vi "Read Display Name.vi"(8 "error in (no error)":errorcluster, 11 "Task in":refnum<class "Task.lvclass">) -> (0 "error out":errorcluster, 2 "Display Name":string, 3 "Task out":refnum<class "Task.lvclass">)   [LabVIEW 2017, in "Task Interface.lvlib" / "Task.lvclass"]
uses:
  Task.lvclass
  Task.lvclass/Task.ctl
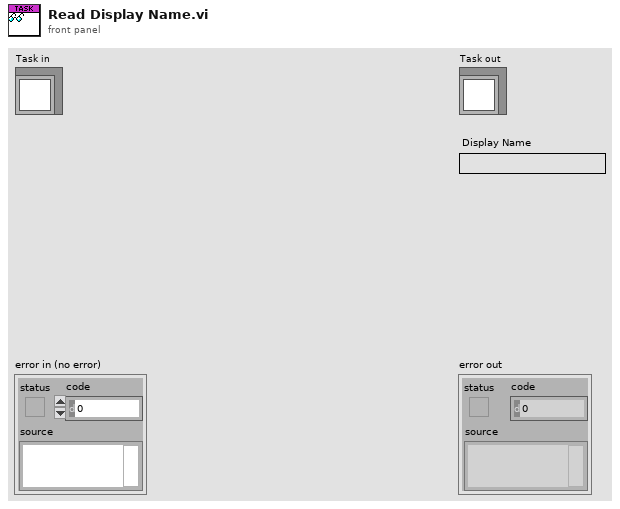
[diagram p1: front panel]
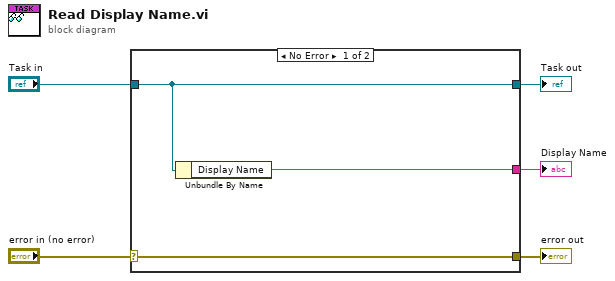
[diagram p0: block diagram]
diagram:
  n1 = case shown="No Error" "error in (no error)" {
    selector: "error in (no error)" -> [w8 w9]
    tunnel: [w8 w9] -> w4
    tunnel: [w7 w10] -> w2
    tunnel: "Task in" -> [w7 w10]
    tunnel: [w6 _] -> w1
    frame No Error {
      n2 = Unbundle By Name(w7) -> ("Display Name"=w6:string)
    }
    frame Error {
    }
  }
  "error out" <- w4
  "Task out" <- w2
  "Display Name" <- w1
